vi "Template.Async.vi"(10 "Parameters":variant, 11 "Process":refnum<class "Process.lvclass">) -> ()   [LabVIEW 2026, in "Template Plugin.lvlib" / "Template.lvclass"]
uses:
  Template.lvclass
  Template.lvclass/Template.ctl
  <userlib>/NIVS Inline Async API (Express)/_VS Inline Async API (Express)/Process/Process.lvclass
  <userlib>/NIVS Inline Async API (Express)/_Data Access Engine (Express)/Data Access Engine (Express)/Data Access Engine (Express).lvclass
  <userlib>/NIVS Inline Async API (Express)/_Data Access Engine (Express)/Data Access Engine (Express)/Methods/Write.Lookup.vi
  <userlib>/NIVS Inline Async API (Express)/_Data Access Engine (Express)/Data Access Engine (Express)/Methods/Read.Lookup.vi
  <userlib>/NIVS Inline Async API (Express)/_Data Access Engine (Express)/Data Access Engine (Express)/Methods/Read.Data.vi
  <userlib>/NIVS Inline Async API (Express)/_Data Access Engine (Express)/Data Access Engine (Express)/Methods/Write.Data.vi
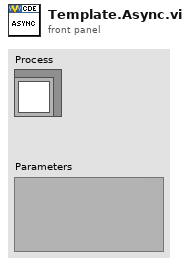
[diagram p1: front panel]
types:
  T1 = typedef "Data Access Engine (Express).lvlib/Data Access Engine (Express).lvclass/Write.DVR.ctl" = refnum<data-value>
  T2 = typedef "Data Access Engine (Express).lvlib/Data Access Engine (Express).lvclass/Read.DVR.ctl" = refnum<data-value>
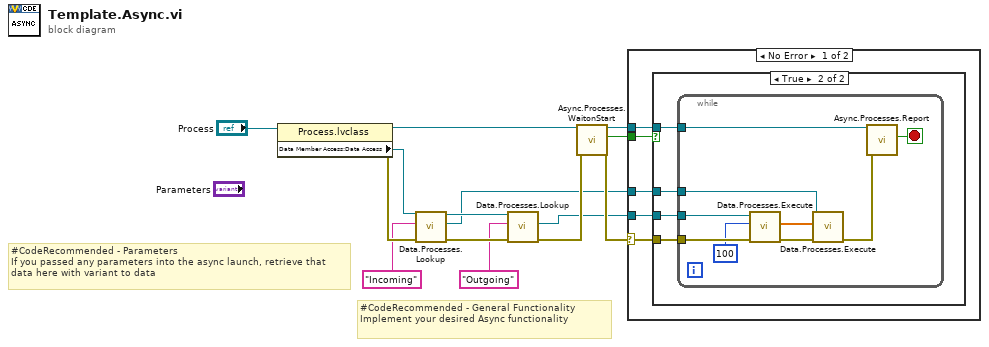
[diagram p0: block diagram]
diagram:
  # "#CodeRecommended - Parameters\nIf you passed any parameters into the async launch, retrieve that\ndata here with variant to data"
  # "#CodeRecommended - General Functionality\nImplement your desired Async functionality"
  n1 = property class="Process.lvclass"(reference="Process") -> (reference out=w7:refnum<class "Process.lvclass">, error out=w11:errorcluster, "Data Member Access:Data Access"=w9:refnum<class "Data Access Engine (Express).lvclass">)  [unwired: 1 in]
  n2 = call-poly <userlib>:"Data.Processes.Lookup.vi"("error in"=w11, "Name"="Incoming", "Data Access API in"=w9) -> ("error out"=w12:errorcluster, "Ref"=w4:T1, "Data Access API out"=w8:refnum<class "Data Access Engine (Express).lvclass">)  [unwired: 5 in, 1 out]
  n3 = call-poly <userlib>:"Data.Processes.Lookup.vi"("error in"=w12, "Name"="Outgoing", "Data Access API in"=w8) -> ("error out"=w14:errorcluster, "Ref"=w5:T2)  [unwired: 5 in, 2 out]
  n4 = call <userlib>:"Async.Processes.WaitonStart.vi"("error in"=w14, "Process in"=w7) -> ("error out"=w13:errorcluster, "Execute"=w6:bool, "Process out"=w3:refnum<class "Process.lvclass">)  [unwired: 7 in]
  n5 = case shown="No Error" w13 {
    selector: w13 -> [w19 _]
    tunnel: w6 -> [w18 _]
    tunnel: w5 -> [w17 _]
    tunnel: w4 -> [w16 _]
    tunnel: w3 -> [w15 _]
    frame No Error {
      n6 = case shown="True" w18 {
        tunnel: w19 -> [_ w23]
        tunnel: w17 -> [_ w22]
        tunnel: w16 -> [_ w21]
        tunnel: w15 -> [_ w20]
        frame False {
        }
        frame True {
          n7 = while {
            tunnel: w23 -> [w32]
            tunnel: w22 -> [w29]
            tunnel: w21 -> [w27]
            tunnel: w20 -> [w25]
            stop <- w24 stop-if-true
            n8 = call-poly <userlib>:"Data.Processes.Execute.vi"("error in"=w32, "timeout ms"=100, "Ref"=w29) -> ("error out"=w31:errorcluster, "Values"=w26:dbl[])  [unwired: 6 in, 1 out]
            n9 = call-poly <userlib>:"Data.Processes.Execute.vi"("error in"=w31, "Values"=w26, "Ref"=w27) -> ("error out"=w30:errorcluster)  [unwired: 8 in]
            n10 = call <userlib>:"Async.Processes.Report.vi"("error in"=w30, "Process in"=w25) -> ("Stop"=w24:bool)  [unwired: 8 in, 1 out]
          }
        }
      }
    }
    frame Error {
    }
  }
